vi "DDSSequence_Ethernet.vi"() -> ()   [LabVIEW 2016]
uses:
  <vilib>/regexp/Match Regular Expression.xnode
panel:
  in  "DDS Slot":u8
  out "Connected":bool
  out "read buffer 2":string
  out "error out 2":errorcluster={"status"=TRUE, "code"=-1073807343, "source"="Property Node (arg 1) in VISA Configure Serial Port (Instr).vi->FlexDDS-NG_USB_VISA_Open.vi->DDSSequence.vi"}
  out "return count 2":u32
  out "Successful":bool
  out "error out 3":errorcluster
  out "data out":string
  in  "error in (no error)":errorcluster
  in  "Freqeuncy (MHz)":dbl[][](array[numeric])=[[1.0, 2.0, 2.0, 1.0, 0.5, 0.0]]
  in  "Power":dbl[][](array[numeric])=[[1.0, 0.0, 0.5, 0.0, 1.0, 0.0]]
  out "Instruction String Slot 2":string="dds 0 reset\rdcp 0 spi:CFR2=0x1000080\rdcp 0 spi:STP0=0x418937\rdcp 0 wait::BNC_IN_A_RISING\rdcp 0 update:u\rdcp 0 spi:STP0=0x3FFF000000418937\rdcp 0 wait:0h:\rdcp 0 update:u\r\rdcp 0 spi:STP0=0x83126F\rdcp 0 wait:62500h:\rdcp 0 update:u\r\rdcp 0 spi:STP0=0x3FFF00000083126F\rdcp 0 wait:31250h:\rdcp 0 update:u\r\rdcp 0 spi:STP0=0x418937\rdcp 0 wait:62500h:\rdcp 0 update:u\r\rdcp 0 spi:DRL=0xFFFC000000000000\rdcp 0 spi:DRSS=0x28F5C29028F5C29\rdcp 0 spi:DRR=0x1F401F4\rdcp 0 spi:CFR2=0x280080\rdcp 0 wait:62500h:\rdcp 0 update:u+d\rdcp 0 wait:125000h:\rdcp 0 update:-d\rdcp 0 spi:CFR2=0x1200080\rdcp 0 spi:STP0=0x418937\rdcp 0 wait:62500h:\rdcp 0 update:u\rdcp 0 start\rdds 1 reset\rdcp 1 spi:CFR2=0x1000080\rdcp 1 spi:STP0=0x418937\rdcp 1 wait::BNC_IN_A_RISING\rdcp 1 update:u\rdcp 1 spi:STP0=0x3FFF000000418937\rdcp 1 wait:0h:\rdcp 1 update:u\r\rdcp 1 spi:STP0=0x83126F\rdcp 1 wait:62500h:\rdcp 1 update:u\r\rdcp 1 spi:STP0=0x200000000083126F\rdcp 1 wait:31250h:\rdcp 1 update:u\r\rdcp 1 spi:STP0=0x418937\rdcp 1 wait:62500h:\rdcp 1 update:u\r\rdcp 1 spi:DRL=0xFFFC000000000000\rdcp 1 spi:DRSS=0x28F5C29028F5C29\rdcp 1 spi:DRR=0x1F401F4\rdcp 1 spi:CFR2=0x280080\rdcp 1 wait:62500h:\rdcp 1 update:u+d\rdcp 1 wait:125000h:\rdcp 1 update:-d\rdcp 1 spi:CFR2=0x1200080\rdcp 1 spi:STP0=0x418937\rdcp 1 wait:62500h:\rdcp 1 update:u\rdcp 1 start\r\r"
  in  "Freqeuncy (MHz)  3":dbl[][](array[numeric])=[[1.0, 2.0, 2.0, 1.0, 0.5, 0.0]]
  in  "Power  3":dbl[][](array[numeric])=[[1.0, 0.0, 1.0, 0.0, 1.0, 0.0]]
  in  "Freqeuncy (MHz)  2":dbl[][](array[numeric])=[[1.0, 2.0, 2.0, 1.0, 0.5, 0.0]]
  in  "Power  2":dbl[][](array[numeric])=[[1.0, 0.0, 0.5, 0.0, 1.0, 0.0]]
  out "Instruction String Slot 1":string="dds 0 reset\rdcp 0 spi:CFR2=0x1000080\rdcp 0 spi:STP0=0x418937\rdcp 0 wait::BNC_IN_A_RISING\rdcp 0 update:u\rdcp 0 spi:STP0=0x3FFF000000418937\rdcp 0 wait:0h:\rdcp 0 update:u\r\rdcp 0 spi:STP0=0x83126F\rdcp 0 wait:62500h:\rdcp 0 update:u\r\rdcp 0 spi:STP0=0x3FFF00000083126F\rdcp 0 wait:31250h:\rdcp 0 update:u\r\rdcp 0 spi:STP0=0x418937\rdcp 0 wait:62500h:\rdcp 0 update:u\r\rdcp 0 spi:DRL=0xFFFC000000000000\rdcp 0 spi:DRSS=0x28F5C29028F5C29\rdcp 0 spi:DRR=0x1F401F4\rdcp 0 spi:CFR2=0x280080\rdcp 0 wait:62500h:\rdcp 0 update:u+d\rdcp 0 wait:125000h:\rdcp 0 update:-d\rdcp 0 spi:CFR2=0x1200080\rdcp 0 spi:STP0=0x418937\rdcp 0 wait:62500h:\rdcp 0 update:u\rdcp 0 start\rdds 1 reset\rdcp 1 spi:CFR2=0x1000080\rdcp 1 spi:STP0=0x418937\rdcp 1 wait::BNC_IN_A_RISING\rdcp 1 update:u\rdcp 1 spi:STP0=0x3FFF000000418937\rdcp 1 wait:0h:\rdcp 1 update:u\r\rdcp 1 spi:STP0=0x83126F\rdcp 1 wait:62500h:\rdcp 1 update:u\r\rdcp 1 spi:STP0=0x200000000083126F\rdcp 1 wait:31250h:\rdcp 1 update:u\r\rdcp 1 spi:STP0=0x418937\rdcp 1 wait:62500h:\rdcp 1 update:u\r\rdcp 1 spi:DRL=0xFFFC000000000000\rdcp 1 spi:DRSS=0x28F5C29028F5C29\rdcp 1 spi:DRR=0x1F401F4\rdcp 1 spi:CFR2=0x280080\rdcp 1 wait:62500h:\rdcp 1 update:u+d\rdcp 1 wait:125000h:\rdcp 1 update:-d\rdcp 1 spi:CFR2=0x1200080\rdcp 1 spi:STP0=0x418937\rdcp 1 wait:62500h:\rdcp 1 update:u\rdcp 1 start\r\r"
  in  "No of  active time blocks":dbl=4.0
  in  "Freqeuncy (MHz) 2":dbl[][](array[numeric])=[[1.0, 2.0, 2.0, 1.0, 0.5, 0.0]]
  in  "Duration (ms)":dbl[][](array[numeric])=[[0.5, 0.25, 0.5, 1.0, 2.0, 1.0]]
  in  "Power 2":dbl[][](array[numeric])=[[1.0, 0.0, 1.0, 0.0, 1.0, 0.0]]
  out "return count":u32=1275
  out "error out":errorcluster={"status"=TRUE, "code"=-1073807339, "source"="VISA Read in DDSSequence.vi"}
  out "read buffer":string
  # "DDS 0"
  # "DDS 1"
  # "DDS 2"
  # "DDS 3"
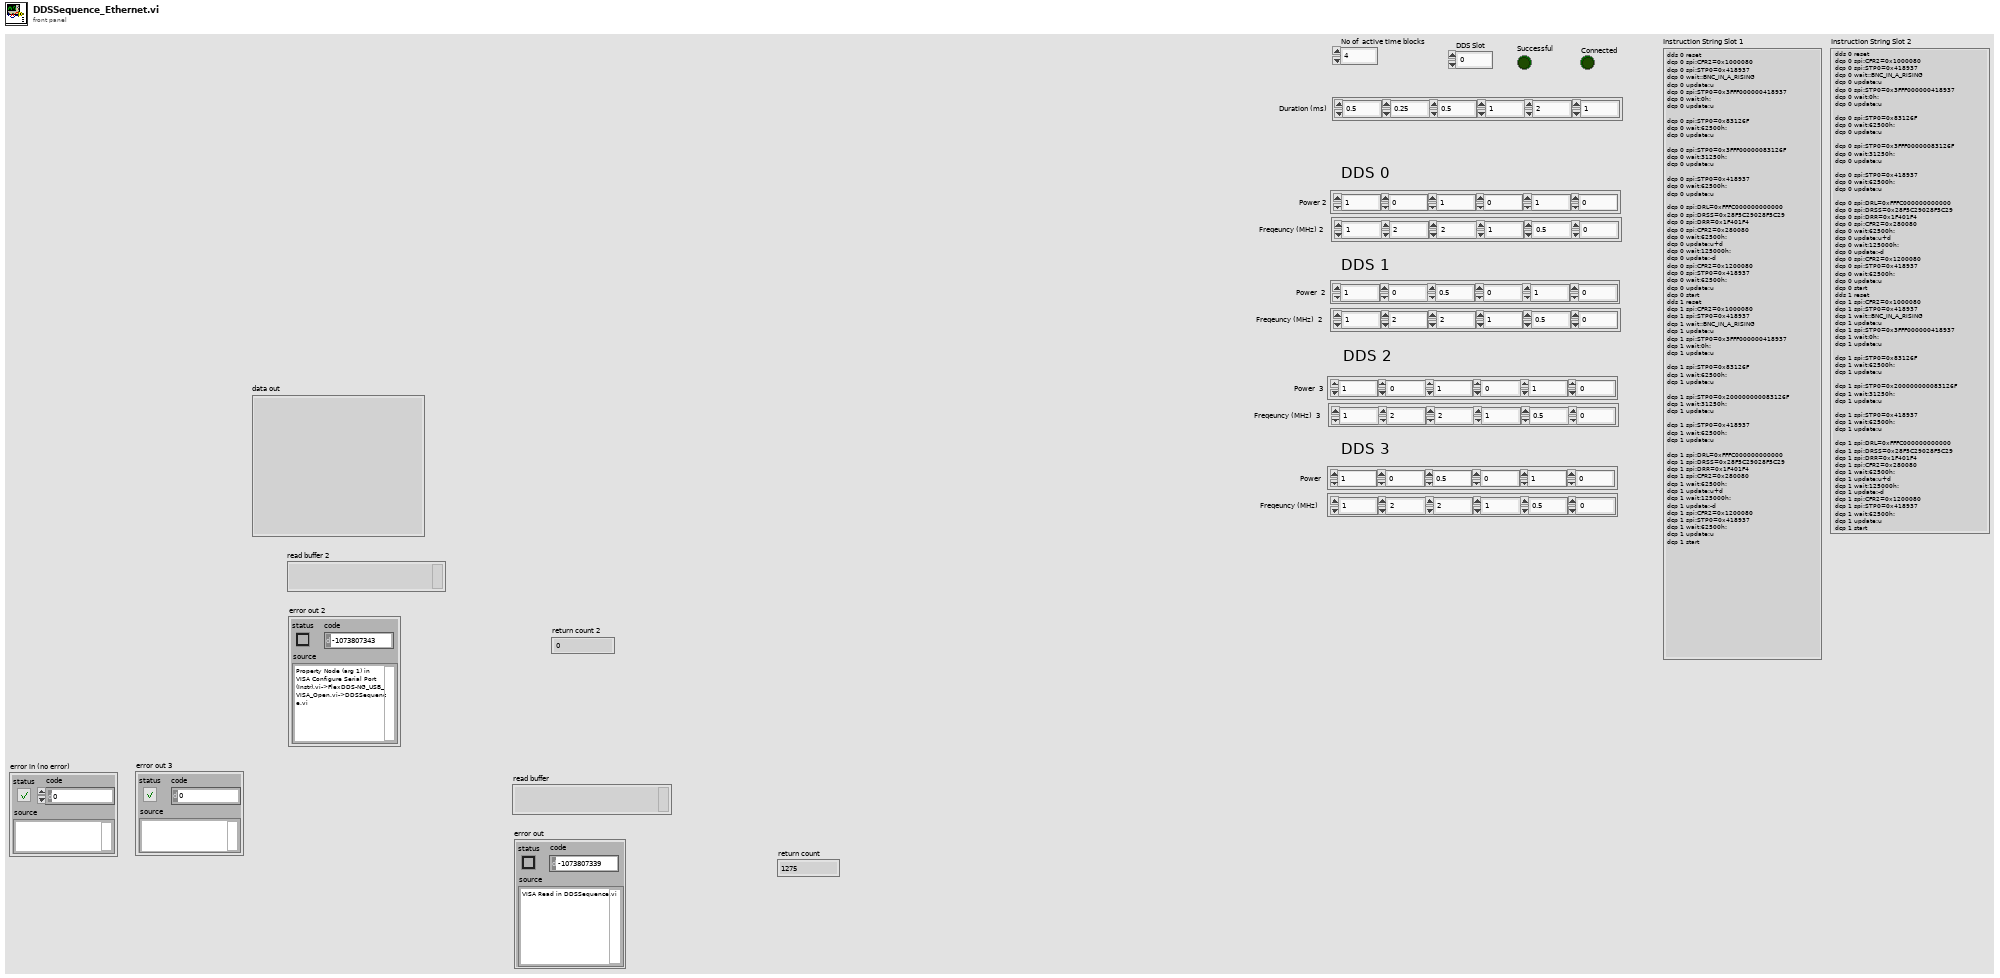
[diagram p1: front panel]
types:
  T1 = enum32{"Channel 0", "Channel 1", "Both channels"}
  T2 = enum16{"Standard", "Buffered", "CRLF", "Immediate"}
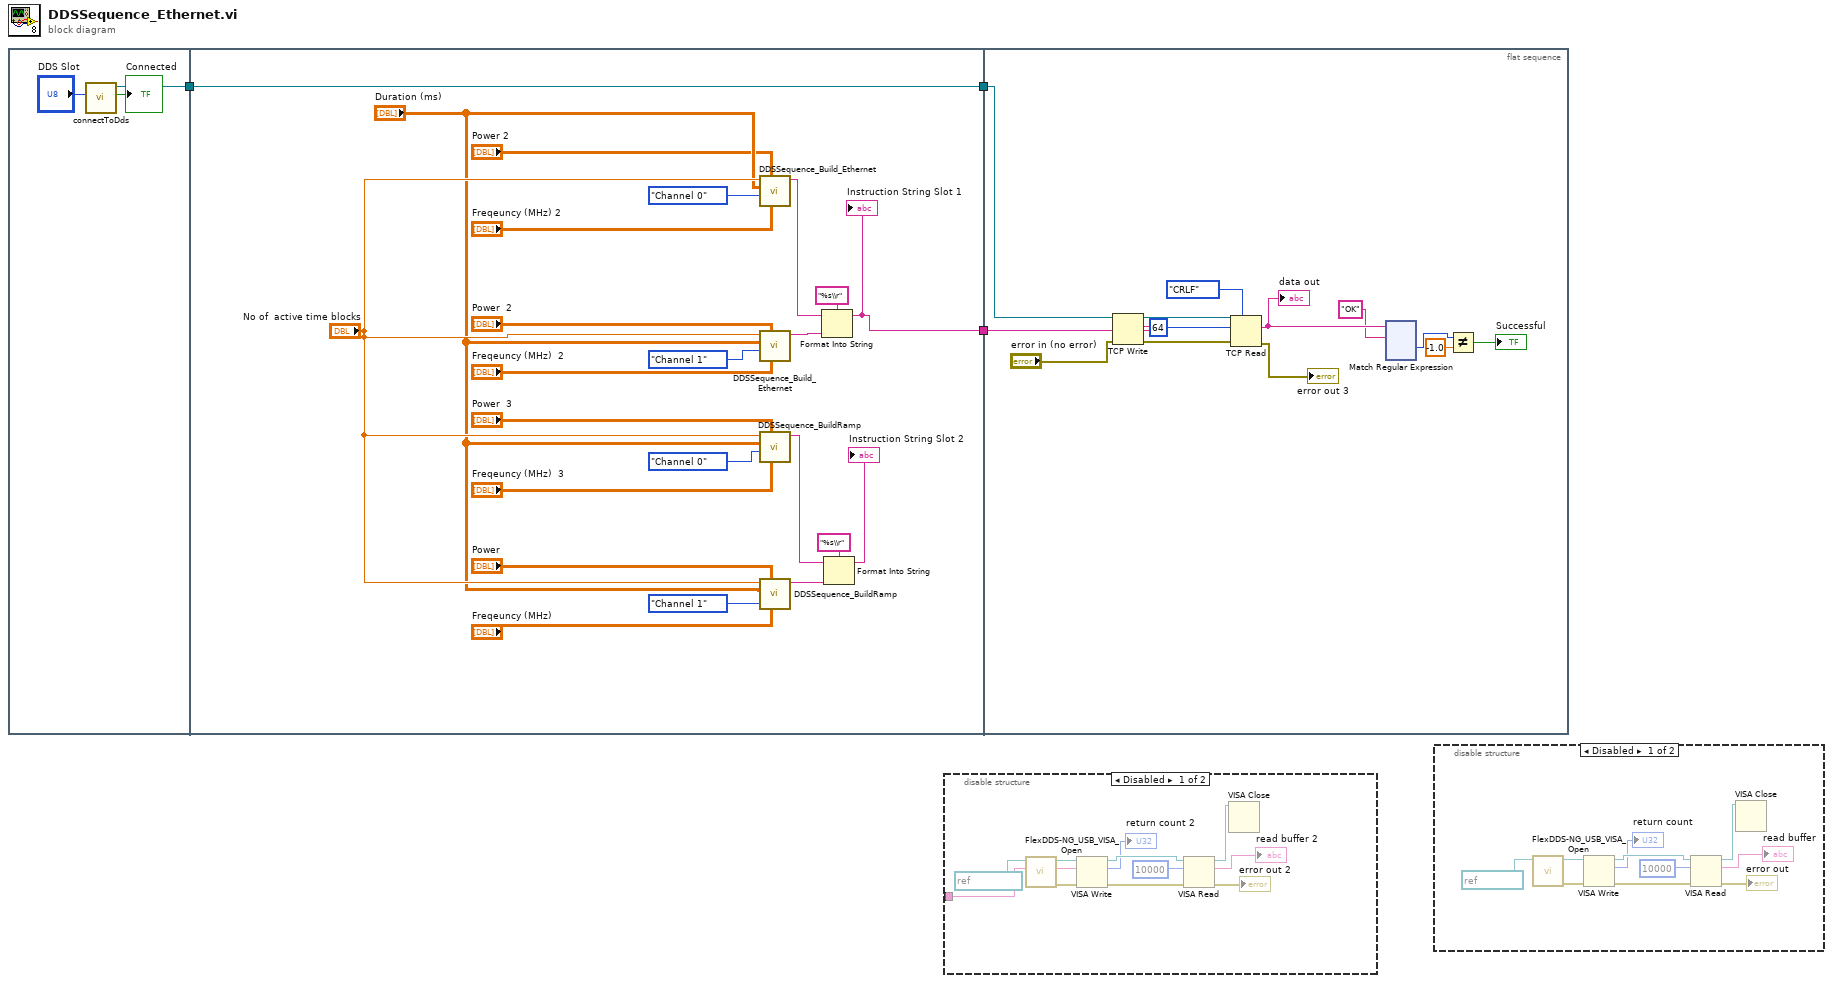
[diagram p0: block diagram]
diagram:
  n1 = flat-sequence {
    tunnel: [w6] -> w3
    tunnel: w3 -> [w8]
    tunnel: [w8] -> w2
    tunnel: [w7] -> w1
    tunnel: w2 -> [w31]
    tunnel: w1 -> [w30]
    frame #0 {
      n2 = call "connectToDds.vi"("DDS Slot"="DDS Slot") -> ("Connected"=→"Connected":bool, "connection ID"=w6:refnum<k5>)  [unwired: 8 in, 1 out]
    }
    frame #1 {
      n3 = call "DDSSequence_Build_Ethernet.vi"("Freqeuncy (MHz)"="Freqeuncy (MHz) 2", "Power"="Power 2", "Channels"=T1."Channel 0", "Duration (ms)"="Duration (ms)", "No of  active time blocks"="No of  active time blocks") -> ("appended instruction string"=w24:string)  [unwired: 6 in]
      n4 = call "DDSSequence_Build_Ethernet.vi"("Freqeuncy (MHz)"="Freqeuncy (MHz)  2", "Power"="Power  2", "Channels"=T1."Channel 1", "Duration (ms)"="Duration (ms)", "No of  active time blocks"="No of  active time blocks") -> ("appended instruction string"=w20:string)  [unwired: 6 in]
      n5 = call "DDSSequence_BuildRamp.vi"("Freqeuncy (MHz)"="Freqeuncy (MHz)  3", "Power"="Power  3", "Channels"=T1."Channel 0", "Duration (ms)"="Duration (ms)", "No of  active time blocks"="No of  active time blocks") -> ("appended instruction string"=w16:string)  [unwired: 6 in]
      n6 = call "DDSSequence_BuildRamp.vi"("Freqeuncy (MHz)"="Freqeuncy (MHz)", "Power"="Power", "Channels"=T1."Channel 1", "Duration (ms)"="Duration (ms)", "No of  active time blocks"="No of  active time blocks") -> ("appended instruction string"=w28:string)  [unwired: 6 in]
      n7 = Format Into String(format string="%s\\r", initial string=w24, w20) -> (resulting string=w7:string)  [unwired: 1 in, 1 out]
      "Instruction String Slot 1" <- w7
      n8 = Format Into String(format string="%s\\r", initial string=w16, w28) -> (resulting string=→"Instruction String Slot 2":string)  [unwired: 1 in, 1 out]
    }
    frame #2 {
      n9 = TCP Write(connection ID=w31, data in=w30, error in (no error)="error in (no error)") -> (connection ID out=w35:refnum<k5>, error out=w37:errorcluster)  [unwired: 1 in, 1 out]
      n10 = TCP Read(connection ID=w35, bytes to read=64, error in (no error)=w37, 7:T2."CRLF" ("mode (standard)")) -> (data out=w41:string, error out=→"error out 3":errorcluster)  [unwired: 1 in, 1 out]
      "data out" <- w41
      n11 = xnode "Match Regular Expression"("input string"=w41, "regular expression"="OK") -> ("offset past match"=w40:i32)  [unwired: 4 in, 4 out]
      n12 = Not Equal?(x=w40, y=-1.0) -> (x != y?=→"Successful":bool)
    }
  }
  n13 = disable-structure shown="Disabled" {
    disable-tunnel: _ -> [w157 _]
    frame Disabled {
      n14 = call "FlexDDS-NG_USB_VISA_Open.vi"("FlexDDS-NG USB VISA resource name (COM)"=refnum<visa-resource-name> "COM11") -> ("error out"=w159:errorcluster, "FlexDDS-NG USB VISA resource name out"=w160:refnum<visa-resource-name>)  [unwired: 9 in]
      n15 = VISA Write(VISA resource name=w160, write buffer=w157, error in (no error)=w159) -> (VISA resource name out=w164:refnum<visa-resource-name>, return count=→"return count 2":u32, error out=w162:errorcluster)
      n16 = VISA Read(VISA resource name=w164, byte count=u32 10000, error in (no error)=w162) -> (VISA resource name out=w167:refnum<visa-resource-name>, read buffer=→"read buffer 2":string, error out=→"error out 2":errorcluster)  [unwired: 1 out]
      n17 = VISA Close(VISA resource name=w167) -> ()  [unwired: 1 in, 1 out]
    }
    frame Enabled {
    }
  }
  n18 = disable-structure shown="Disabled" {
    frame Disabled {
      n19 = call "FlexDDS-NG_USB_VISA_Open.vi"("FlexDDS-NG USB VISA resource name (COM)"=refnum<visa-resource-name> "COM1") -> ("error out"=w169:errorcluster, "FlexDDS-NG USB VISA resource name out"=w170:refnum<visa-resource-name>)  [unwired: 9 in]
      n20 = VISA Write(VISA resource name=w170, error in (no error)=w169) -> (VISA resource name out=w174:refnum<visa-resource-name>, return count=→"return count":u32, error out=w172:errorcluster)  [unwired: 1 in]
      n21 = VISA Read(VISA resource name=w174, byte count=u32 10000, error in (no error)=w172) -> (VISA resource name out=w177:refnum<visa-resource-name>, read buffer=→"read buffer":string, error out=→"error out":errorcluster)  [unwired: 1 out]
      n22 = VISA Close(VISA resource name=w177) -> ()  [unwired: 1 in, 1 out]
    }
    frame Enabled {
    }
  }
